vi "Turn Smother.vi"(1 "Ignore Deceleration":bool, 2 "Ignore Acceleration":bool, 3 "input cluster":T2) -> (0 "Angular Accelerations":T1)   [LabVIEW 2020]
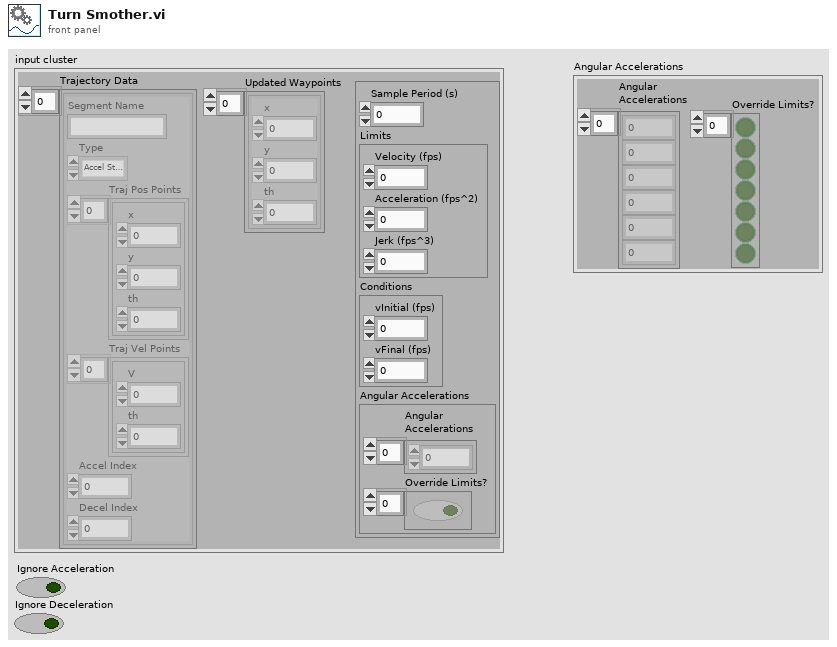
[diagram p1: front panel]
types:
  T1 = cluster{"Angular \nAccelerations":dbl[], "Override Limits?":bool[]}
  T2 = cluster{"Trajectory Data":cluster{"Segment Name":string, "Type":enum16{"Accel Straight", "Const Straight", "Blend", "Circle"}, "Traj Pos Points":cluster{"x":dbl, "y":dbl, "th":dbl}[], "Traj Vel Points":cluster{"V":dbl, "th":dbl}[], "Accel Index":i32, "Decel Index":i32}[], "Updated Waypoints":cluster{"x":dbl, "y":dbl, "th":dbl}[], cluster{"Sample Period (s)":dbl, "Limits":cluster{"Velocity (fps)":dbl, "Acceleration (fps^2)":dbl, "Jerk (fps^3)":dbl}, "Conditions":cluster{"vInitial (fps)":dbl, "vFinal (fps)":dbl}, "Angular Accelerations":cluster{"Angular \nAccelerations":dbl[], "Override Limits?":bool[]}}}
  T3 = cluster{"Segment Name":string, "Type":enum16{"Accel Straight", "Const Straight", "Blend", "Circle"}, "Traj Pos Points":cluster{"x":dbl, "y":dbl, "th":dbl}[], "Traj Vel Points":cluster{"V":dbl, "th":dbl}[], "Accel Index":i32, "Decel Index":i32}[]
  T4 = cluster{"Sample Period (s)":dbl, "Limits":cluster{"Velocity (fps)":dbl, "Acceleration (fps^2)":dbl, "Jerk (fps^3)":dbl}, "Conditions":cluster{"vInitial (fps)":dbl, "vFinal (fps)":dbl}, "Angular Accelerations":cluster{"Angular \nAccelerations":dbl[], "Override Limits?":bool[]}}
  T5 = cluster{"Velocity (fps)":dbl, "Acceleration (fps^2)":dbl, "Jerk (fps^3)":dbl}
  T6 = cluster{"vInitial (fps)":dbl, "vFinal (fps)":dbl}
  T7 = cluster{"Segment Name":string, "Type":enum16{"Accel Straight", "Const Straight", "Blend", "Circle"}, "Traj Pos Points":cluster{"x":dbl, "y":dbl, "th":dbl}[], "Traj Vel Points":cluster{"V":dbl, "th":dbl}[], "Accel Index":i32, "Decel Index":i32}
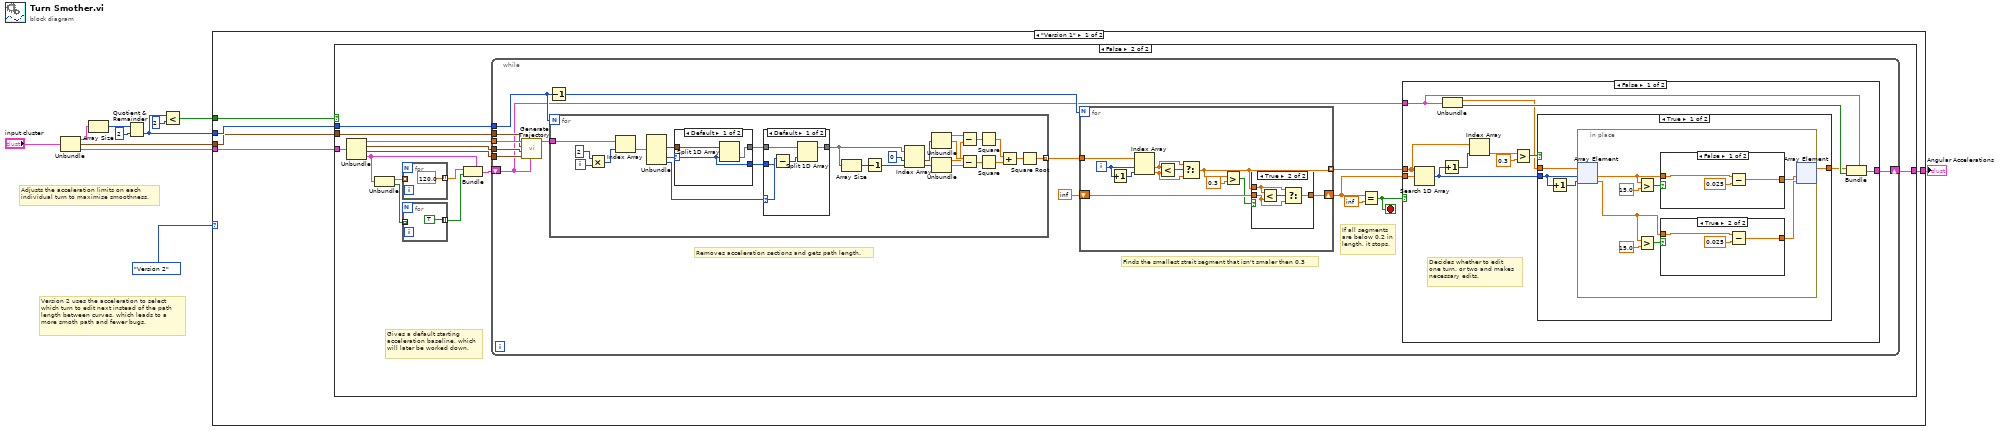
[diagram p0: block diagram]
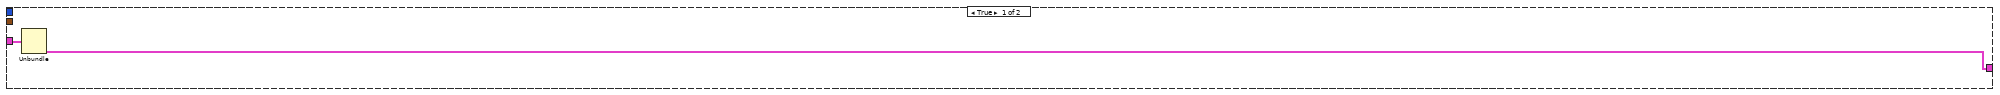
[diagram p2: hidden frame]
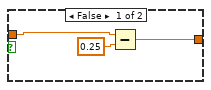
[diagram p5: hidden frame]
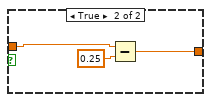
[diagram p6: hidden frame]
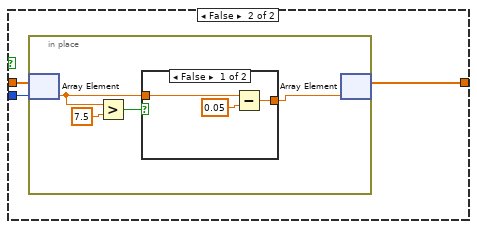
[diagram p7: hidden frame]
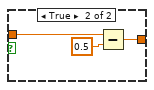
[diagram p8: hidden frame]
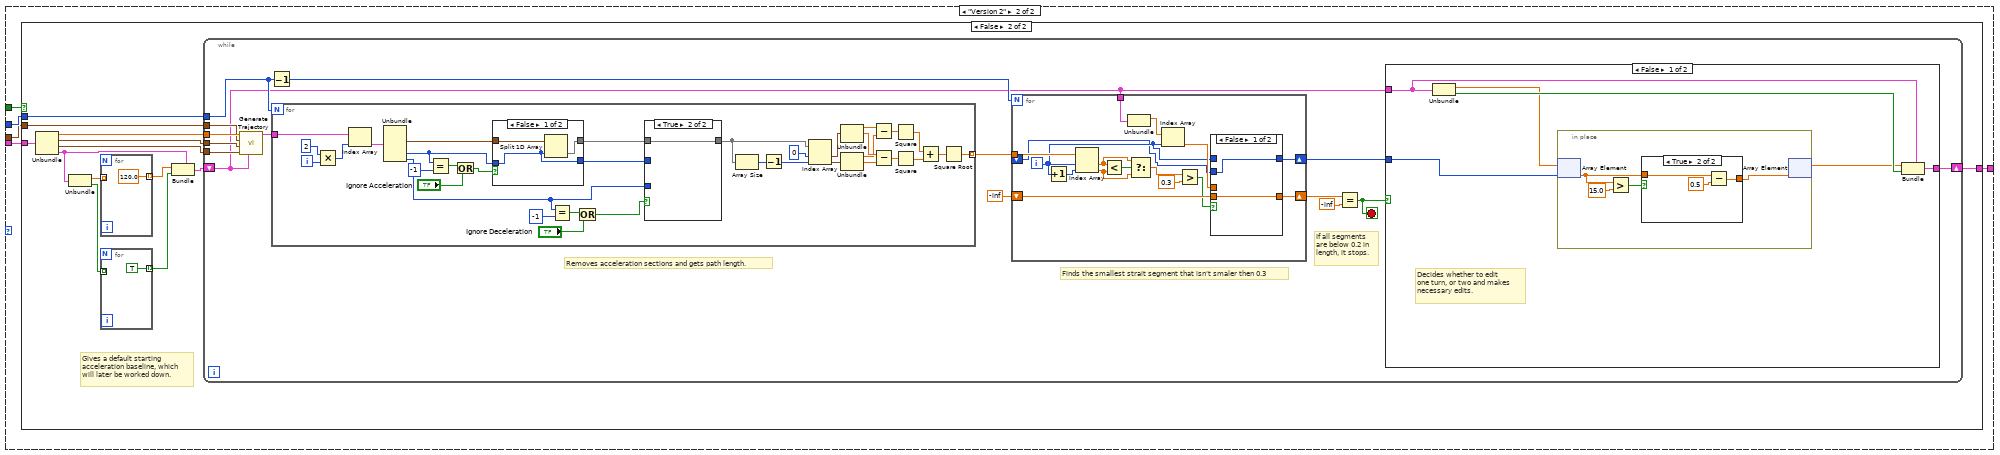
[diagram p11: hidden frame]
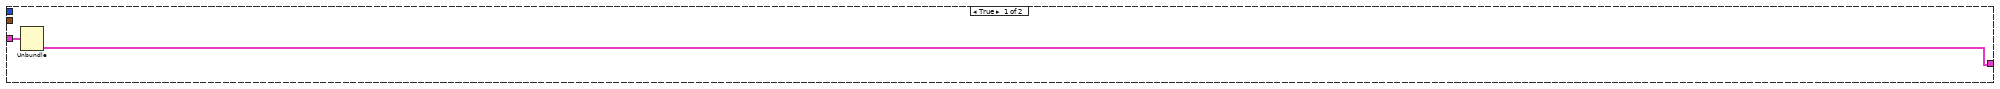
[diagram p12: hidden frame]
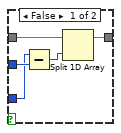
[diagram p13: hidden frame]
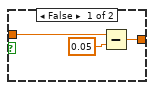
[diagram p15: hidden frame]
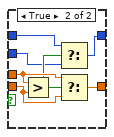
[diagram p17: hidden frame]
diagram:
  # "Version 2 uses the acceleration to select\nwhich turn to edit next instead of the path \nlength between curves, which leads to a \nmore smoth path and fewer bugs."
  # "Adjusts the acceleration limits on each \nindividual turn to maximise smoothness."
  n1 = Unbundle("input cluster") -> ("Trajectory Data"=w4:T3, "Updated Waypoints"=w3:cluster{"x":dbl, "y":dbl, "th":dbl}[], w5:T4)
  n2 = Array Size(array=w4) -> (size(s)=w11:i32)
  n3 = Quotient & Remainder(x=w11, y=2) -> (floor(x/y)=w7:i32)  [unwired: 1 out]
  n4 = Less?(x=w7, y=2) -> (x < y?=w6:bool)
  n5 = case shown="\"Version 1\"" enum16{"Version 2", "Version 1"}."Version 2" {
    tunnel: w7 -> [w16 w155]
    tunnel: w6 -> [w15 w154]
    tunnel: w5 -> [w14 w153]
    tunnel: w3 -> [w13 w152]
    tunnel: [w12 w151] -> w2
    frame "Version 1" {
      n6 = case shown="False" w15 {
        tunnel: w16 -> [_ w25]
        tunnel: [w18 w24] -> w12
        tunnel: w14 -> [w17 w23]
        tunnel: w13 -> [_ w21]
        frame True {
          n7 = Unbundle(w17) -> ("Angular Accelerations"=w18:T1)  [unwired: 3 out]
        }
        frame False {
          # "Gives a default starting \nacceleration baseline, which\nwill later be worked down."
          n8 = Unbundle(w23) -> ("Sample Period (s)"=w22:dbl, "Limits"=w20:T5, "Conditions"=w19:T6, "Angular Accelerations"=w31:T1)
          n9 = Unbundle(w31) -> ("Angular \nAccelerations"=w30:dbl[], "Override Limits?"=w29:bool[])
          n10 = for {
            tunnel: w30 -> [_] mode=indexing
            tunnel: [120.0] -> w28 mode=indexing
          }
          n11 = for {
            tunnel: w29 -> [_] mode=indexing
            tunnel: [TRUE] -> w27 mode=indexing
          }
          n12 = Bundle(cluster=w31, "Angular \nAccelerations"=w28, "Override Limits?"=w27) -> (w26:T1)
          n13 = while {
            shift-right: [w43] -> w24
            shift-left: w26 -> [w34]
            tunnel: w25 -> [w40]
            tunnel: w22 -> [w38]
            tunnel: w21 -> [w37]
            tunnel: w20 -> [w36]
            tunnel: w19 -> [w35]
            stop <- w46 stop-if-true
            # "If all segments\nare below 0.2 in\nlength, it stops."
            # "Removes acceleration sections and gets path length."
            # "Finds the smallest strait segment that isn't smaler then 0.3"
            n14 = call "Generate Trajectory.vi"("Angular Accelerations"=w34, "Conditions"=w35, "Limits"=w36, "WayPoints"=w37, "Sample Period (s)"=w38) -> ("Trajectory Data"=w39:T3)  [unwired: 2 in, 4 out]
            n15 = Decrement(x=w40) -> (x-1=w41:i32)
            n16 = for {
              N: w40 -> [_]
              tunnel: w39 -> [w70]
              tunnel: [w47] -> w42 mode=indexing
              i -> [w72]
              n17 = Multiply(x=2, y=w72) -> (x*y=w69:i32)
              n18 = Index Array(array=w70, index=w69) -> (element=w68:T7)
              n19 = Unbundle(w68) -> ("Traj Pos Points"=w48:cluster{"x":dbl, "y":dbl, "th":dbl}[], "Accel Index"=w65:i32, "Decel Index"=w64:i32)  [unwired: 3 out]
              n20 = case shown="Default" w65 {
                selector: w65 -> [w79 _]
                tunnel: w48 -> [w81 w82]
                tunnel: [w80 w82] -> w67
                tunnel: [w79 _] -> w66
                frame Default {
                  n21 = Split 1D Array(array=w81, index=w79) -> (second subarray=w80:cluster{"x":dbl, "y":dbl, "th":dbl}[])  [unwired: 1 out]
                }
                frame -1 {
                }
              }
              n22 = case shown="Default" w64 {
                selector: w64 -> [w75 _]
                tunnel: w67 -> [w77 w78]
                tunnel: [w76 w78] -> w62
                tunnel: w66 -> [w74 _]
                frame Default {
                  n23 = Subtract(x=w75, y=w74) -> (x-y=w73:i32)
                  n24 = Split 1D Array(array=w77, index=w73) -> (first subarray=w76:cluster{"x":dbl, "y":dbl, "th":dbl}[])  [unwired: 1 out]
                }
                frame -1 {
                }
              }
              n25 = Array Size(array=w62) -> (size(s)=w61:i32)
              n26 = Decrement(x=w61) -> (x-1=w60:i32)
              n27 = Index Array(array=w62, index #1=0 ("index"), index #2=w60) -> (element #1=w50:cluster{"x":dbl, "y":dbl, "th":dbl}, element #2=w49:cluster{"x":dbl, "y":dbl, "th":dbl})
              n28 = Unbundle(w50) -> ("x"=w51:dbl, "y"=w53:dbl)  [unwired: 1 out]
              n29 = Unbundle(w49) -> ("x"=w52:dbl, "y"=w54:dbl)  [unwired: 1 out]
              n30 = Subtract(x=w51, y=w52) -> (x-y=w55:dbl)
              n31 = Subtract(x=w53, y=w54) -> (x-y=w56:dbl)
              n32 = Square(x=w55) -> (x^2=w57:dbl)
              n33 = Square(x=w56) -> (x^2=w58:dbl)
              n34 = Add(x=w57, y=w58) -> (x+y=w59:dbl)
              n35 = Square Root(x=w59) -> (sqrt(x)=w47:dbl)
            }
            n36 = for {
              N: w41 -> [_]
              tunnel: w42 -> [w143]
              shift-right: [w137] -> w45
              shift-left: inf -> [w136]
              tunnel: [w134] -> w44 mode=indexing
              i -> [w142]
              n37 = Increment(x=w142) -> (x+1=w141:i32)
              n38 = Index Array(array=w143, index #1=w142, index #2=w141) -> (element #1=w138:dbl, element #2=w139:dbl)
              n39 = Less?(x=w138, y=w139) -> (x < y?=w140:bool)
              n40 = Select(t=w138, s=w140, f=w139) -> (s? t:f=w134:dbl)
              n41 = Greater?(x=w134, y=0.3) -> (0:w135:bool)
              n42 = case shown="True" w135 {
                tunnel: [w144 w147] -> w137
                tunnel: w136 -> [w144 w146]
                tunnel: w134 -> [_ w145]
                frame False {
                }
                frame True {
                  n43 = Less?(x=w145, y=w146) -> (x < y?=w148:bool)
                  n44 = Select(t=w145, s=w148, f=w146) -> (s? t:f=w147:dbl)
                }
              }
            }
            n45 = Equal?(x=w45, y=inf) -> (x = y?=w46:bool)
            n46 = case shown="False" w46 {
              tunnel: w45 -> [w94 _]
              tunnel: w44 -> [w90 _]
              tunnel: w34 -> [w92 w132]
              tunnel: [w91 w132] -> w43
              frame False {
                # "Decides whether to edit\none turn, or two and makes\nnecessary edits."
                n47 = Search 1D Array(1D array=w90, element=w94) -> (index of element=w84:i32)  [unwired: 1 in]
                n48 = Increment(x=w84) -> (x+1=w89:i32)
                n49 = Unbundle(w92) -> ("Angular \nAccelerations"=w85:dbl[], "Override Limits?"=w93:bool[])
                n50 = Index Array(array=w90, index=w89) -> (element=w88:dbl)
                n51 = Greater?(x=w88, y=0.3) -> (0:w86:bool)
                n52 = case shown="True" w86 {
                  tunnel: w85 -> [w98 w121]
                  tunnel: w84 -> [w96 w120]
                  tunnel: [w97 w119] -> w83
                  frame True {
                    n53 = Increment(x=w96) -> (x+1=w95:i32)
                    n54 = in-place {
                      n55 = in-place-array #1(w98, w96, w95) -> (w103:dbl, w100:dbl)
                      n56 = Greater?(x=w103, y=15.0) -> (0:w104:bool)
                      n57 = Greater?(x=w100, y=15.0) -> (0:w102:bool)
                      n58 = case shown="False" w104 {
                        tunnel: [w114 w117] -> w106
                        tunnel: w103 -> [w115 w116]
                        frame False {
                          n59 = Subtract(x=w115, y=0.025) -> (x-y=w114:dbl)
                        }
                        frame True {
                          n60 = Subtract(x=w116, y=0.25) -> (x-y=w117:dbl)
                        }
                      }
                      n61 = case shown="True" w102 {
                        tunnel: [w108 w111] -> w99
                        tunnel: w100 -> [w109 w110]
                        frame False {
                          n62 = Subtract(x=w109, y=0.25) -> (x-y=w108:dbl)
                        }
                        frame True {
                          n63 = Subtract(x=w110, y=0.025) -> (x-y=w111:dbl)
                        }
                      }
                      n64 = in-place-array #1(w106, w99) -> (w97:dbl[])  [unwired: 2 out]
                    }
                  }
                  frame False {
                    n65 = in-place {
                      n66 = in-place-array #2(w121, w120) -> (w122:dbl)
                      n67 = Greater?(x=w122, y=7.5) -> (0:w123:bool)
                      n68 = case shown="False" w123 {
                        tunnel: [w127 w130] -> w125
                        tunnel: w122 -> [w128 w129]
                        frame False {
                          n69 = Subtract(x=w128, y=0.05) -> (x-y=w127:dbl)
                        }
                        frame True {
                          n70 = Subtract(x=w129, y=0.5) -> (x-y=w130:dbl)
                        }
                      }
                      n71 = in-place-array #2(w125) -> (w119:dbl[])  [unwired: 1 out]
                    }
                  }
                }
                n72 = Bundle(cluster=w92, "Angular \nAccelerations"=w83, "Override Limits?"=w93) -> (w91:T1)
              }
              frame True {
              }
            }
          }
        }
      }
    }
    frame "Version 2" {
      n73 = case shown="False" w154 {
        tunnel: w155 -> [_ w164]
        tunnel: [w157 w163] -> w151
        tunnel: w153 -> [w156 w162]
        tunnel: w152 -> [_ w160]
        frame True {
          n74 = Unbundle(w156) -> ("Angular Accelerations"=w157:T1)  [unwired: 3 out]
        }
        frame False {
          # "Gives a default starting \nacceleration baseline, which\nwill later be worked down."
          n75 = Unbundle(w162) -> ("Sample Period (s)"=w161:dbl, "Limits"=w159:T5, "Conditions"=w158:T6, "Angular Accelerations"=w170:T1)
          n76 = Unbundle(w170) -> ("Angular \nAccelerations"=w169:dbl[], "Override Limits?"=w168:bool[])
          n77 = for {
            tunnel: w169 -> [_] mode=indexing
            tunnel: [120.0] -> w167 mode=indexing
          }
          n78 = for {
            tunnel: w168 -> [_] mode=indexing
            tunnel: [TRUE] -> w166 mode=indexing
          }
          n79 = Bundle(cluster=w170, "Angular \nAccelerations"=w167, "Override Limits?"=w166) -> (w165:T1)
          n80 = while {
            shift-right: [w183] -> w163
            shift-left: w165 -> [w172]
            tunnel: w164 -> [w180]
            tunnel: w161 -> [w178]
            tunnel: w160 -> [w177]
            tunnel: w159 -> [w176]
            tunnel: w158 -> [w175]
            stop <- w185 stop-if-true
            # "If all segments\nare below 0.2 in\nlength, it stops."
            # "Removes acceleration sections and gets path length."
            # "Finds the smallest strait segment that isn't smaler then 0.3"
            n81 = call "Generate Trajectory.vi"("Angular Accelerations"=w172, "Conditions"=w175, "Limits"=w176, "WayPoints"=w177, "Sample Period (s)"=w178) -> ("Trajectory Data"=w179:T3)  [unwired: 2 in, 4 out]
            n82 = Decrement(x=w180) -> (x-1=w181:i32)
            n83 = for {
              N: w180 -> [_]
              tunnel: w179 -> [w217]
              tunnel: [w196] -> w182 mode=indexing
              i -> [w219]
              n84 = Multiply(x=2, y=w219) -> (x*y=w216:i32)
              n85 = Index Array(array=w217, index=w216) -> (element=w215:T7)
              n86 = Unbundle(w215) -> ("Traj Pos Points"=w197:cluster{"x":dbl, "y":dbl, "th":dbl}[], "Accel Index"=w193:i32, "Decel Index"=w186:i32)  [unwired: 3 out]
              n87 = Equal?(x=w193, y=-1) -> (x = y?=w194:bool)
              n88 = Or(x=w194, y="Ignore Acceleration") -> (x .or. y?=w192:bool)
              n89 = case shown="False" w192 {
                tunnel: w197 -> [w228 w229]
                tunnel: [w227 w229] -> w214
                tunnel: [w226 _] -> w213
                tunnel: w193 -> [w226 _]
                frame False {
                  n90 = Split 1D Array(array=w228, index=w226) -> (second subarray=w227:cluster{"x":dbl, "y":dbl, "th":dbl}[])  [unwired: 1 out]
                }
                frame True {
                }
              }
              n91 = Equal?(x=w186, y=-1) -> (x = y?=w189:bool)
              n92 = Or(x=w189, y="Ignore Deceleration") -> (x .or. y?=w187:bool)
              n93 = case shown="True" w187 {
                tunnel: w214 -> [w224 w225]
                tunnel: [w223 w225] -> w211
                tunnel: w213 -> [w222 _]
                tunnel: w186 -> [w220 _]
                frame False {
                  n94 = Subtract(x=w220, y=w222) -> (x-y=w221:i32)
                  n95 = Split 1D Array(array=w224, index=w221) -> (first subarray=w223:cluster{"x":dbl, "y":dbl, "th":dbl}[])  [unwired: 1 out]
                }
                frame True {
                }
              }
              n96 = Array Size(array=w211) -> (size(s)=w210:i32)
              n97 = Decrement(x=w210) -> (x-1=w209:i32)
              n98 = Index Array(array=w211, index #1=0 ("index"), index #2=w209) -> (element #1=w199:cluster{"x":dbl, "y":dbl, "th":dbl}, element #2=w198:cluster{"x":dbl, "y":dbl, "th":dbl})
              n99 = Unbundle(w199) -> ("x"=w200:dbl, "y"=w202:dbl)  [unwired: 1 out]
              n100 = Unbundle(w198) -> ("x"=w201:dbl, "y"=w203:dbl)  [unwired: 1 out]
              n101 = Subtract(x=w200, y=w201) -> (x-y=w204:dbl)
              n102 = Subtract(x=w202, y=w203) -> (x-y=w205:dbl)
              n103 = Square(x=w204) -> (x^2=w206:dbl)
              n104 = Square(x=w205) -> (x^2=w207:dbl)
              n105 = Add(x=w206, y=w207) -> (x+y=w208:dbl)
              n106 = Square Root(x=w208) -> (sqrt(x)=w196:dbl)
            }
            n107 = for {
              N: w181 -> [_]
              tunnel: w182 -> [w262]
              shift-right: [w257] -> w184
              shift-left: -inf -> [w256]
              tunnel: w172 -> [w252]
              shift-right: [w248] -> w171
              shift-left: _ -> [w247]
              i -> [w249]
              n108 = Increment(x=w249) -> (x+1=w261:i32)
              n109 = Index Array(array=w262, index #1=w249, index #2=w261) -> (element #1=w258:dbl, element #2=w259:dbl)
              n110 = Less?(x=w258, y=w259) -> (x < y?=w260:bool)
              n111 = Unbundle(w252) -> ("Angular \nAccelerations"=w251:dbl[])  [unwired: 1 out]
              n112 = Select(t=w258, s=w260, f=w259) -> (s? t:f=w254:dbl)
              n113 = Index Array(array=w251, index=w249) -> (element=w250:dbl)
              n114 = Greater?(x=w254, y=0.3) -> (0:w255:bool)
              n115 = case shown="False" w255 {
                tunnel: [w264 w271] -> w257
                tunnel: w256 -> [w264 w270]
                tunnel: w250 -> [_ w269]
                tunnel: w249 -> [_ w267]
                tunnel: [w263 w265] -> w248
                tunnel: w247 -> [w263 w266]
                frame False {
                }
                frame True {
                  n116 = Greater?(x=w269, y=w270) -> (0:w268:bool)
                  n117 = Select(t=w267, s=w268, f=w266) -> (s? t:f=w265:i32)
                  n118 = Select(t=w269, s=w268, f=w270) -> (s? t:f=w271:dbl)
                }
              }
            }
            n119 = Equal?(x=w184, y=-inf) -> (x = y?=w185:bool)
            n120 = case shown="False" w185 {
              tunnel: w172 -> [w234 w246]
              tunnel: [w233 w246] -> w183
              tunnel: w171 -> [w230 _]
              frame False {
                # "Decides whether to edit\none turn, or two and makes\nnecessary edits."
                n121 = Unbundle(w234) -> ("Angular \nAccelerations"=w232:dbl[], "Override Limits?"=w235:bool[])
                n122 = in-place {
                  n123 = in-place-array #3(w232, w230) -> (w236:dbl)
                  n124 = Greater?(x=w236, y=15.0) -> (0:w237:bool)
                  n125 = case shown="True" w237 {
                    tunnel: [w241 w244] -> w239
                    tunnel: w236 -> [w242 w243]
                    frame False {
                      n126 = Subtract(x=w242, y=0.05) -> (x-y=w241:dbl)
                    }
                    frame True {
                      n127 = Subtract(x=w243, y=0.5) -> (x-y=w244:dbl)
                    }
                  }
                  n128 = in-place-array #3(w239) -> (w231:dbl[])  [unwired: 1 out]
                }
                n129 = Bundle(cluster=w234, "Angular \nAccelerations"=w231, "Override Limits?"=w235) -> (w233:T1)
              }
              frame True {
              }
            }
          }
        }
      }
    }
  }
  "Angular Accelerations" <- w2
